vi "AlliGator Compute Weighted Phasor Plot Statistics (Core).vi"(6 "Phasor Frequency":dbl[unit], 8 "error in (no error)":errorcluster, 9 "Intensity Array":dbl[](array[numeric]), 10 "s Array":dbl[](array[numeric]), 11 "g Array":dbl[](array[numeric])) -> (0 "error out":errorcluster, 1 "Result String":string, 2 "Effective # Elements":i32, 3 "Phasor Plot Statistics":T1, 4 "All defined?":bool)   [LabVIEW 2021, in "AlliGator Phasor Graph.lvlib"]
uses:
  AlliGator Phasor Graph.lvlib
  AlliGator Phasor Plot Statistics.ctl
  Phasor/Phasor (g, s).ctl
  <userlib>/_OpenG.lib/array/array.llb/Delete Elements from 1D Array (DBL)__ogtk.vi
  Phasor/Phasor.lvlib
  Math/Math.lvlib
  <userlib>/_OpenG.lib/array/array.llb/openg_array.lvlib
  Arrays/Arrays.lvlib
  Phasor Ratio/AlliGator Phasor Ratio.lvlib
panel:
  # "see the License on the block diagram (Ctrl+E or Window:Show Block Diagram)"
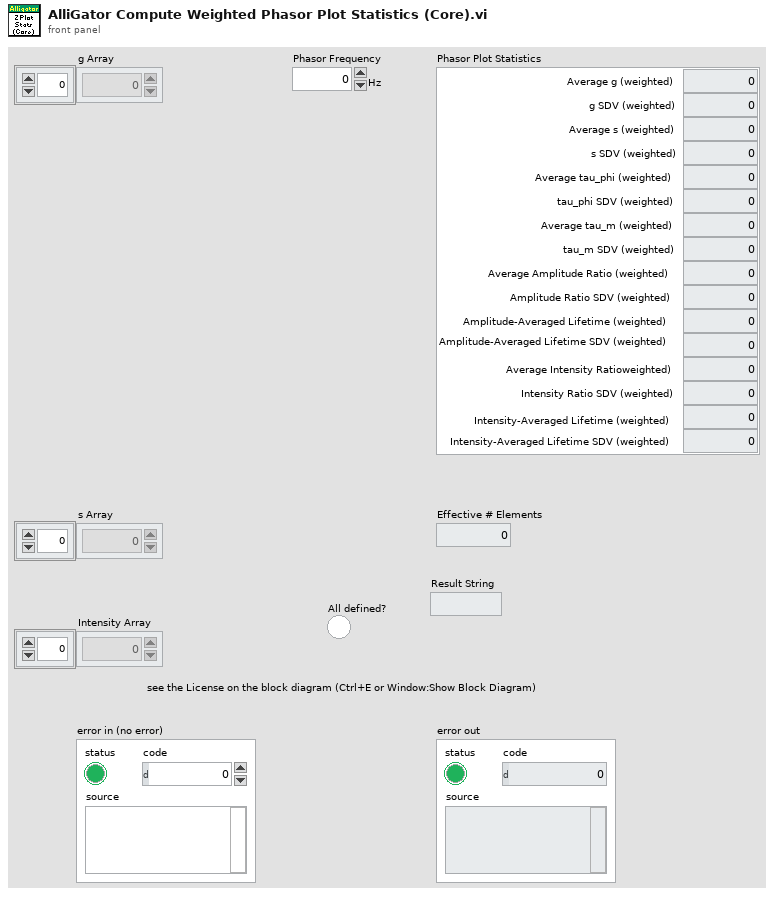
[diagram p1: front panel]
types:
  T1 = typedef "AlliGator Phasor Graph.lvlib/AlliGator Phasor Plot Statistics.ctl" = cluster{"Average g (weighted)":dbl, "g SDV (weighted)":dbl, "Average s (weighted)":dbl, "s SDV (weighted)":dbl, "Average tau_phi (weighted)":dbl, "tau_phi SDV (weighted)":dbl, "Average tau_m (weighted)":dbl, "tau_m SDV (weighted)":dbl, "Average Amplitude Ratio (weighted)":dbl, "Amplitude Ratio SDV (weighted)":dbl, "Amplitude-Averaged Lifetime (weighted)":dbl, "Amplitude-Averaged Lifetime SDV (weighted)":dbl, "Average Intensity Ratioweighted)":dbl, "Intensity Ratio SDV (weighted)":dbl, "Intensity-Averaged Lifetime (weighted)":dbl, "Intensity-Averaged Lifetime SDV (weighted)":dbl}
  T2 = typedef "Phasor.lvlib/Phasor (g, s).ctl" = cluster{"g":dbl, "s":dbl}
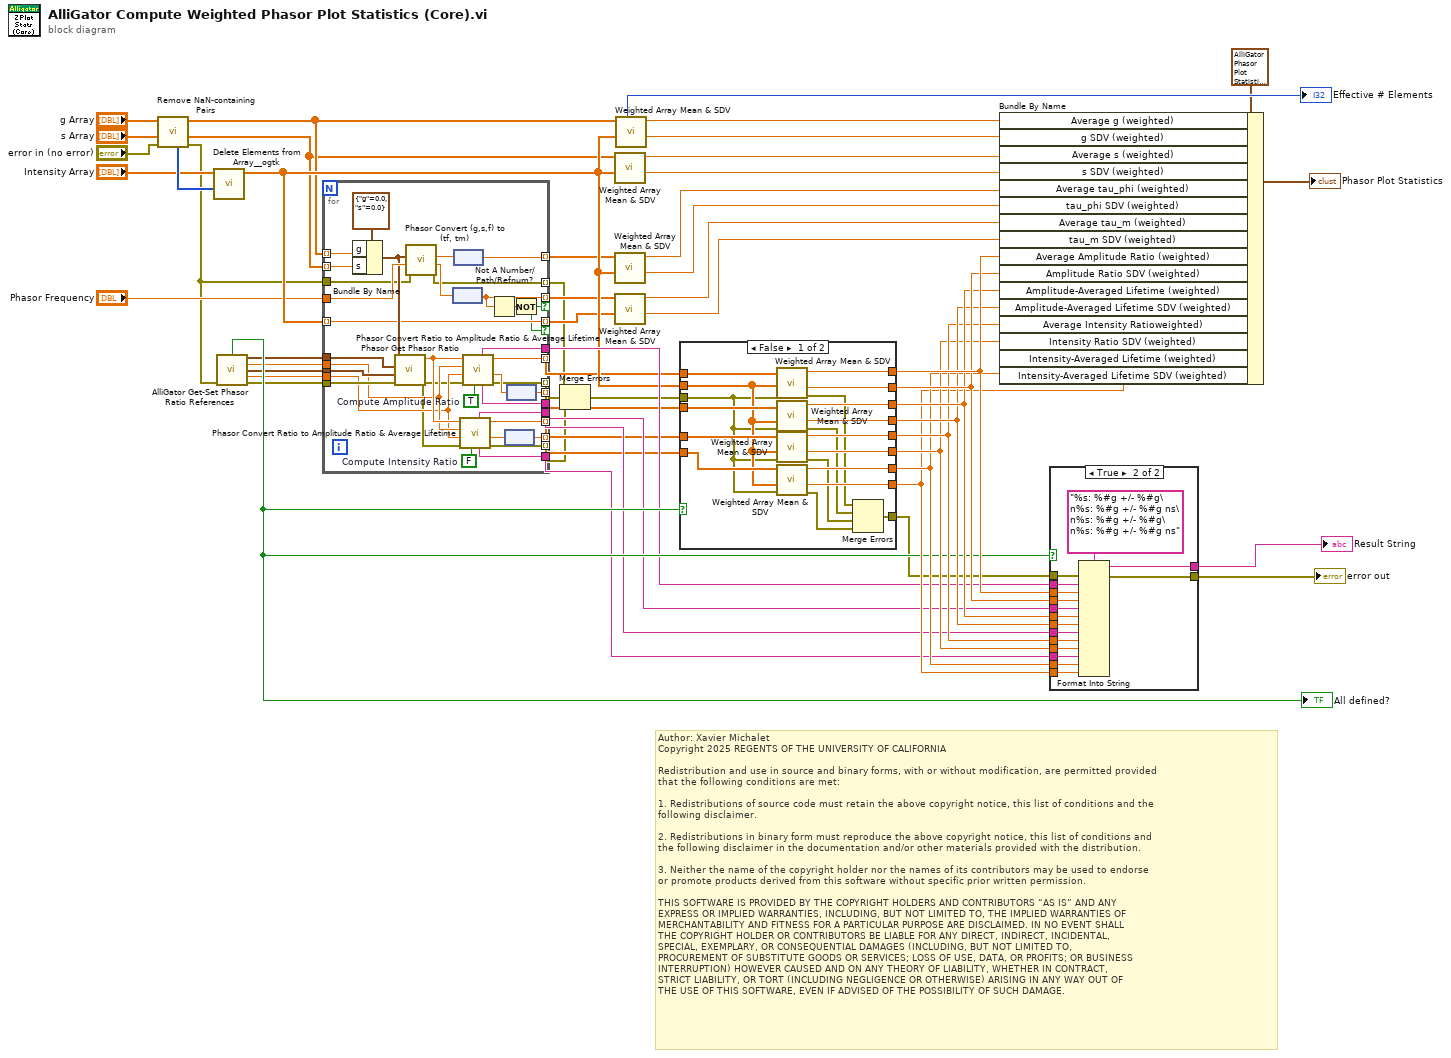
[diagram p0: block diagram]
diagram:
  # "Author: Xavier Michalet\nCopyright 2025 REGENTS OF THE UNIVERSITY OF CALIFORNIA\n\nRedistribution and use in source and binary forms, with or without modification, are permitted provided\nthat the following conditions are met:\n\n1. Redistributions of source code must retain the above copyright notice, this list of conditions and the\nfollowing disclaimer.\n\n2. Redistributions in binary form must reproduce the above copyright notice, this list of conditions and\nthe following disclaimer in the documentation and/or other materials provided with the distribution.\n\n3. Neither the name of the copyright holder nor the names of its contributors may be used to endorse \nor promote products derived from this software without specific prior written permission.\n\nTHIS SOFTWARE IS PROVIDED BY THE COPYRIGHT HOLDERS AND CONTRIBUTORS “AS IS” AND ANY \nEXPRESS OR IMPLIED WARRANTIES, INCLUDING, BUT NOT LIMITED TO, THE IMPLIED WARRANTIES OF\nMERCHANTABILITY AND FITNESS FOR A PARTICULAR PURPOSE ARE DISCLAIMED. IN NO EVENT SHALL\nTHE COPYRIGHT HOLDER OR CONTRIBUTORS BE LIABLE FOR ANY DIRECT, INDIRECT, INCIDENTAL, \nSPECIAL, EXEMPLARY, OR CONSEQUENTIAL DAMAGES (INCLUDING, BUT NOT LIMITED TO, \nPROCUREMENT OF SUBSTITUTE GOODS OR SERVICES; LOSS OF USE, DATA, OR PROFITS; OR BUSINESS\nINTERRUPTION) HOWEVER CAUSED AND ON ANY THEORY OF LIABILITY, WHETHER IN CONTRACT, \nSTRICT LIABILITY, OR TORT (INCLUDING NEGLIGENCE OR OTHERWISE) ARISING IN ANY WAY OUT OF\nTHE USE OF THIS SOFTWARE, EVEN IF ADVISED OF THE POSSIBILITY OF SUCH DAMAGE."
  n1 = call "Remove NaN-containing Pairs.vi"("Error In"="error in (no error)", "Y Array in"="s Array", "X Array in"="g Array") -> ("Error Out"=w7:errorcluster, "Y Array out"=w5:dbl[], "X Array out"=w6:dbl[], "Deleted Elts Indices"=w25:i32[])  [unwired: 4 in, 1 out]
  n2 = call-poly <userlib>:"Delete Elements from Array__ogtk.vi"("indices"=w25, "array"="Intensity Array") -> ("array w/ subset deleted"=w26:dbl[])  [unwired: 8 in, 1 out]
  n3 = call "AlliGator Get-Set Phasor Ratio References.vi"("error in (no error)"=w7) -> ("All defined?"=w34:bool, "Reference Phasor 1"=w17:T2, "Reference Lifetime 1"=w15:dbl[unit], "Reference Phasor 2"=w16:T2, "Reference Lifetime 2"=w14:dbl[unit], "error out"=w19:errorcluster)  [unwired: 7 in, 2 out]
  "All defined?" <- w34
  n4 = for {
    tunnel: w5 -> [w86] mode=indexing
    tunnel: w6 -> [w87] mode=indexing
    tunnel: "Phasor Frequency" -> [w84]
    tunnel: [w85] -> w4 mode=indexing
    tunnel: [w81] -> w3 mode=indexing if=w54
    tunnel: w19 -> [w79]
    tunnel: w16 -> [w78]
    tunnel: w17 -> [w77]
    tunnel: w14 -> [w66]
    tunnel: w15 -> [w67]
    tunnel: [w75] -> w13 mode=indexing
    tunnel: [w74] -> w27
    tunnel: [w70] -> w18 mode=indexing
    tunnel: [w72] -> w12 mode=indexing
    tunnel: [w71] -> w28
    tunnel: [w63] -> w29
    tunnel: [w62] -> w11 mode=indexing
    tunnel: [w60] -> w10 mode=indexing
    tunnel: [w59] -> w8 mode=indexing
    tunnel: [w58] -> w30
    tunnel: w7 -> [w57]
    tunnel: [w56] -> w1 mode=indexing
    tunnel: w26 -> [w55] mode=indexing
    tunnel: [w55] -> w2 mode=indexing if=w54
    w64 = FALSE  # Compute Intensity Ratio
    w69 = TRUE  # Compute Amplitude Ratio
    n5 = Bundle By Name(cluster=T2 {"g"=0.0, "s"=0.0} ("Phasor (g, s)"), "g"=w87, "s"=w86) -> (w76:T2)
    n6 = call "Phasor Get Phasor Ratio.vi"("Error In"=w79, "Reference Phasor 2"=w78, "Reference Phasor 1"=w77, "Phasor"=w76) -> ("Error Out"=w65:errorcluster, "Phasor Ratio (f1)"=w68:dbl)  [unwired: 5 in, 1 out]
    n7 = call "Phasor Convert (g,s,f) to (tf, tm).vi"("Error In"=w57, "Phasor Harmonic Frequency"=w84, "Phasor (g, s)"=w76) -> ("Error Out"=w56:errorcluster, "Modulus Lifetime"=w82:dbl[unit], "Phase Lifetime"=w83:dbl[unit])  [unwired: 6 in]
    n8 = node(w82) -> (w81:dbl)
    n9 = node(w83) -> (w85:dbl)
    n10 = call "Phasor Convert Ratio to Amplitude Ratio & Average Lifetime.vi"("Compute Amplitude Ratio"=w64, "error in (no error)"=w65, "Reference Lifetime 2"=w66, "Reference Lifetime 1"=w67, "Phasor Ratio (f1)"=w68) -> ("error out"=w59:errorcluster, "Average Lifetime"=w61:dbl[unit], "Phasor/Amplitude Ratio"=w62:dbl, "Average Lifetime Caption"=w58:string, "Phasor Ratio Plot Name Suffix"=w63:string)  [unwired: 2 in]
    n11 = call "Phasor Convert Ratio to Amplitude Ratio & Average Lifetime.vi"("Compute Amplitude Ratio"=w69, "error in (no error)"=w65, "Reference Lifetime 2"=w66, "Reference Lifetime 1"=w67, "Phasor Ratio (f1)"=w68) -> ("error out"=w72:errorcluster, "Average Lifetime"=w73:dbl[unit], "Phasor/Amplitude Ratio"=w75:dbl, "Average Lifetime Caption"=w71:string, "Phasor Ratio Plot Name Suffix"=w74:string)  [unwired: 2 in]
    n12 = Not A Number/Path/Refnum?(number/path/refnum=w81) -> (NaN/Path/Refnum?=w80:bool)
    n13 = node(w61) -> (w60:dbl)
    n14 = node(w73) -> (w70:dbl)
    n15 = Not(x=w80) -> (.not. x?=w54:bool)
  }
  n16 = Merge Errors(w1, w12, w8) -> (w9:errorcluster)
  n17 = call "Weighted Array Mean & SDV.vi"("Weight Array"=w26, "Array"=w5) -> ("SDV (weighted)"=w43:dbl, "Average Value (weighted)"=w44:dbl)  [unwired: 4 in, 4 out]
  n18 = call "Weighted Array Mean & SDV.vi"("Weight Array"=w26, "Array"=w4) -> ("SDV (weighted)"=w49:dbl, "Average Value (weighted)"=w48:dbl)  [unwired: 4 in, 4 out]
  n19 = call "Weighted Array Mean & SDV.vi"("Weight Array"=w2, "Array"=w3) -> ("SDV (weighted)"=w51:dbl, "Average Value (weighted)"=w50:dbl)  [unwired: 4 in, 4 out]
  n20 = call "Weighted Array Mean & SDV.vi"("Weight Array"=w26, "Array"=w6) -> ("SDV (weighted)"=w45:dbl, "Average Value (weighted)"=w46:dbl, "Effective # Elements"=→"Effective # Elements":i32)  [unwired: 4 in, 3 out]
  n21 = case shown="False" w34 {
    tunnel: w18 -> [w106 _]
    tunnel: w13 -> [w107 _]
    tunnel: w9 -> [w94 w108]
    tunnel: w11 -> [w105 _]
    tunnel: w10 -> [w104 _]
    tunnel: w26 -> [w103 _]
    tunnel: [w102 _] -> w42
    tunnel: [w101 _] -> w41
    tunnel: [w100 _] -> w40
    tunnel: [w99 _] -> w39
    tunnel: [w98 _] -> w38
    tunnel: [w97 _] -> w37
    tunnel: [w96 _] -> w36
    tunnel: [w95 _] -> w35
    tunnel: [w89 w108] -> w33
    frame False {
      n22 = call "Weighted Array Mean & SDV.vi"("Error In"=w94, "Weight Array"=w103, "Array"=w107) -> ("Error Out"=w93:errorcluster, "SDV (weighted)"=w101:dbl, "Average Value (weighted)"=w102:dbl)  [unwired: 3 in, 3 out]
      n23 = call "Weighted Array Mean & SDV.vi"("Error In"=w94, "Weight Array"=w103, "Array"=w106) -> ("Error Out"=w92:errorcluster, "SDV (weighted)"=w99:dbl, "Average Value (weighted)"=w100:dbl)  [unwired: 3 in, 3 out]
      n24 = call "Weighted Array Mean & SDV.vi"("Error In"=w94, "Weight Array"=w103, "Array"=w105) -> ("Error Out"=w91:errorcluster, "SDV (weighted)"=w97:dbl, "Average Value (weighted)"=w98:dbl)  [unwired: 3 in, 3 out]
      n25 = call "Weighted Array Mean & SDV.vi"("Error In"=w94, "Weight Array"=w103, "Array"=w104) -> ("Error Out"=w90:errorcluster, "SDV (weighted)"=w95:dbl, "Average Value (weighted)"=w96:dbl)  [unwired: 3 in, 3 out]
      n26 = Merge Errors(w93, w92, w91, w90) -> (w89:errorcluster)
    }
    frame True {
    }
  }
  n27 = Bundle By Name(cluster=T1 {"Average g (weighted)"=0.0, "g SDV (weighted)"=0.0, "Average s (weighted)"=0.0, "s SDV (weighted)"=0.0, "Average tau_phi (weighted)"=0.0, "tau_phi SDV (weighted)"=0.0, "Average tau_m (weighted)"=0.0, "tau_m SDV (weighted)"=0.0, "Average Amplitude Ratio (weighted)"=0.0, "Amplitude Ratio SDV (weighted)"=0.0, "Amplitude-Averaged Lifetime (weighted)"=0.0, "Amplitude-Averaged Lifetime SDV (weighted)"=0.0, "Average Intensity Ratioweighted)"=0.0, "Intensity Ratio SDV (weighted)"=0.0, "Intensity-Averaged Lifetime (weighted)"=0.0, "Intensity-Averaged Lifetime SDV (weighted)"=0.0} ("Phasor Plot Statistics"), "Average g (weighted)"=w46, "g SDV (weighted)"=w45, "Average s (weighted)"=w44, "s SDV (weighted)"=w43, "Average tau_phi (weighted)"=w48, "tau_phi SDV (weighted)"=w49, "Average tau_m (weighted)"=w50, "tau_m SDV (weighted)"=w51, "Average Amplitude Ratio (weighted)"=w42, "Amplitude Ratio SDV (weighted)"=w41, "Amplitude-Averaged Lifetime (weighted)"=w40, "Amplitude-Averaged Lifetime SDV (weighted)"=w39, "Average Intensity Ratioweighted)"=w38, "Intensity Ratio SDV (weighted)"=w37, "Intensity-Averaged Lifetime (weighted)"=w36, "Intensity-Averaged Lifetime SDV (weighted)"=w35) -> (→"Phasor Plot Statistics":T1)
  n28 = case shown="True" w34 {
    tunnel: w27 -> [_ w124]
    tunnel: w42 -> [_ w123]
    tunnel: w41 -> [_ w122]
    tunnel: w28 -> [_ w121]
    tunnel: w40 -> [_ w120]
    tunnel: w39 -> [_ w119]
    tunnel: w29 -> [_ w118]
    tunnel: w38 -> [_ w117]
    tunnel: w37 -> [_ w116]
    tunnel: w30 -> [_ w115]
    tunnel: w36 -> [_ w114]
    tunnel: w35 -> [_ w113]
    tunnel: [_ w112] -> w31
    tunnel: [w109 w111] -> w32
    tunnel: w33 -> [w109 w110]
    frame False {
    }
    frame True {
      n29 = Format Into String(format string="%s: %#g +/- %#g\n%s: %#g +/- %#g ns\n%s: %#g +/- %#g\n%s: %#g +/- %#g ns", error in=w110, w124, w123, w122, w121, w120, w119, w118, w117, w116, w115, w114, w113) -> (resulting string=w112:string, error out=w111:errorcluster)  [unwired: 1 in]
    }
  }
  "error out" <- w32
  "Result String" <- w31
